vi "Validate Data Types.vi"(8 "error in (no error)":errorcluster, 11 "Cluster":variant) -> (0 "error out":errorcluster)   [LabVIEW 2020, in "MeasurementLink Measurement Server.lvlib"]
uses:
  MeasurementLink Measurement Server.lvlib
  a8e12af1-21a4-44b4-83f7-8cc59a2476b7.vi
  b0d8a33e-d00a-40db-a7bc-a08db774de9e.vi
  <vilib>/Comparison/Equal/Equal Functor/Equal Functor.lvclass
  <vilib>/Utility/Data Type/NI_Data Type.lvlib
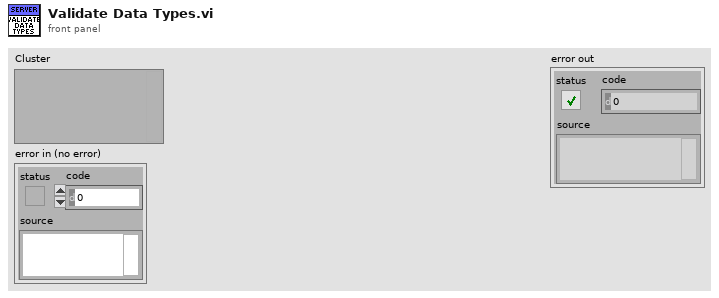
[diagram p1: front panel]
types:
  T1 = typedef "NI_Data Type.lvlib/Data Type.ctl" = enum8{"Invalid Type", "Void", "I8", "I16", "I32", "I64", "U8", "U16", "U32", "U64", "Single Float", "Double Float", "Extended Float", "Single Complex", "Double Complex", "Extended Complex", "Enum U8", "Enum U16", "Enum U32", "Enum U64", "Single Float With Unit", "Double Float With Unit", "Extended Float With Unit", "Single Complex with Unit", "Double Complex with Unit", "Extended Complex with Unit", "Boolean", "String", "Path", "Picture", "Tag", "Array", "Cluster", "Variant", "LV Variant", "Waveform", "Timestamp", "Digital Waveform", "Digital Data", "ExpressData", "Refnum", "External Data", "VI", "Poly VI", "LabVIEW Class Instance", "Fixed Point", "Set Collection", "Map Collection"}
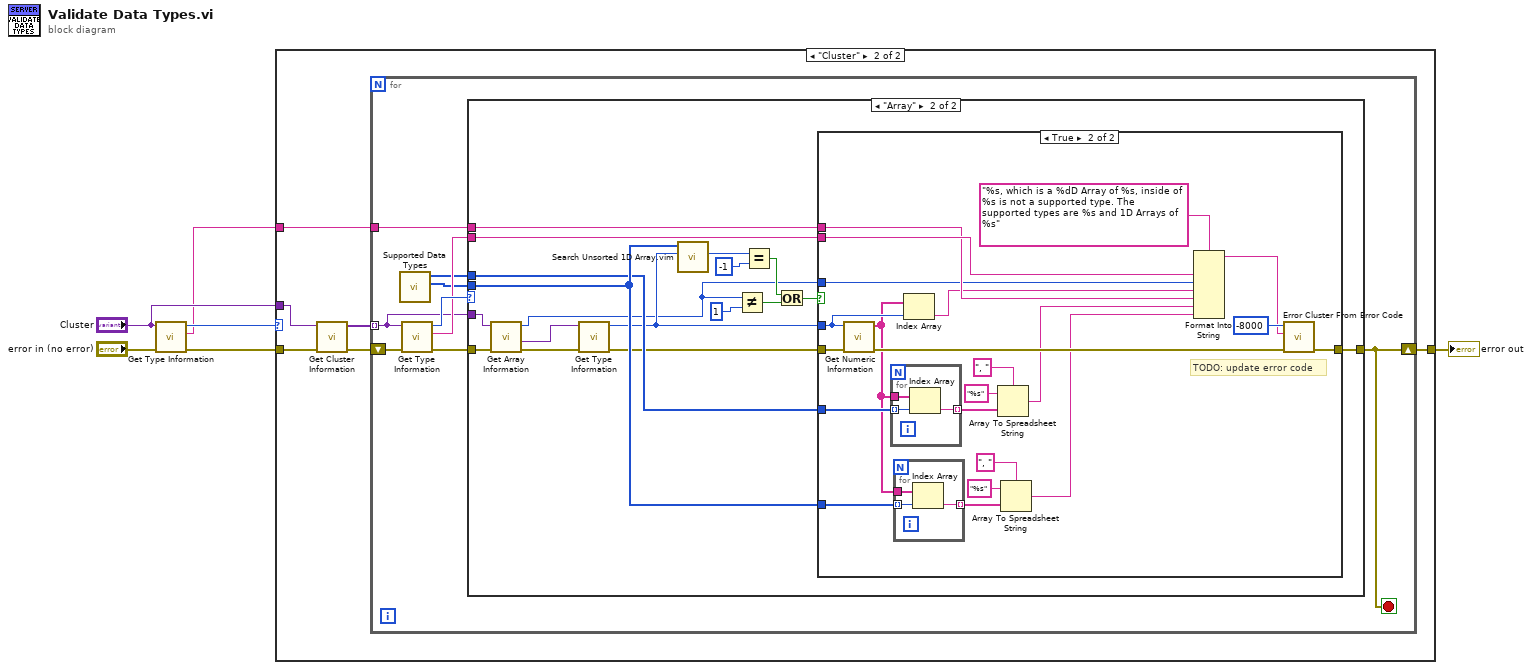
[diagram p0: block diagram]
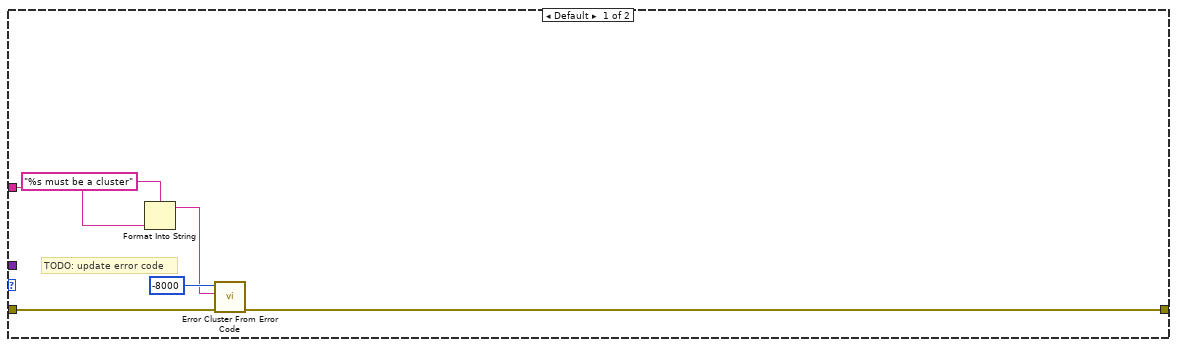
[diagram p2: hidden frame]
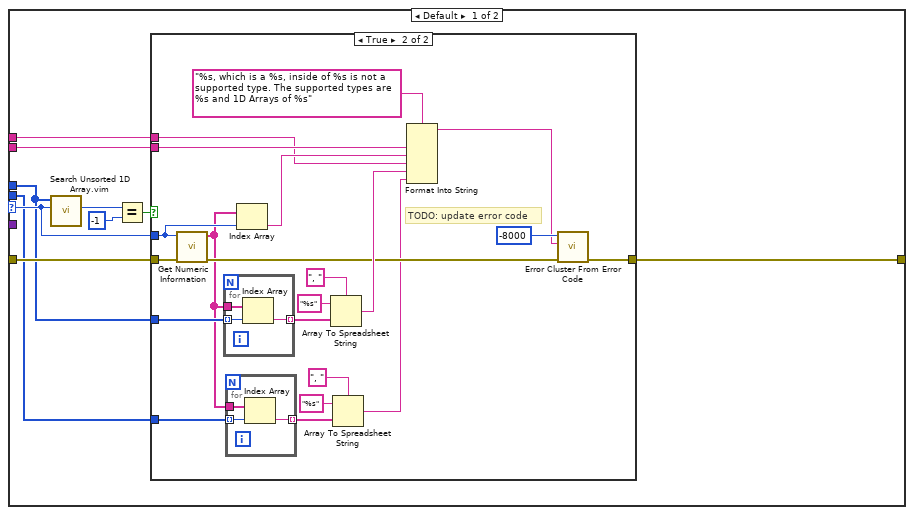
[diagram p3: hidden frame]
diagram:
  n1 = call <vilib>:"Get Type Information.vi"("error in (no error)"="error in (no error)", "variant"="Cluster") -> ("error out"=w6:errorcluster, "name"=w3:string, "type"=w5:T1)  [unwired: 5 in, 2 out]
  n2 = case shown="\"Cluster\"" w5 {
    tunnel: [w11 w13] -> w1
    tunnel: w6 -> [w12 w18]
    tunnel: "Cluster" -> [_ w17]
    tunnel: w3 -> [w8 w14]
    frame Default {
      # "TODO: update error code"
      n3 = Format Into String(format string="%s must be a cluster", w8) -> (resulting string=w7:string)  [unwired: 2 in, 1 out]
      n4 = call <vilib>:"Error Cluster From Error Code.vi"("error in (no error)"=w12, "error message (\"\")"=w7, "error code (0)"=-8000) -> ("error out"=w11:errorcluster)  [unwired: 6 in]
    }
    frame "Cluster" {
      n5 = call <vilib>:"Get Cluster Information.vi"("error in (no error)"=w18, "variant"=w17) -> ("error out"=w16:errorcluster, "cluster elements"=w15:variant[])  [unwired: 8 in]
      n6 = for {
        tunnel: w15 -> [w22] mode=indexing
        tunnel: w14 -> [w25]
        shift-right: [w21] -> w13
        shift-left: w16 -> [w27]
        stop <- w21 stop-if-true
        n7 = call "Supported Data Types.vi"() -> ("Supported Types In Arrays"=w19:T1[], "Supported Types"=w20:T1[])  [unwired: 10 in]
        n8 = call <vilib>:"Get Type Information.vi"("error in (no error)"=w27, "variant"=w22) -> ("error out"=w23:errorcluster, "name"=w24:string, "type"=w26:T1)  [unwired: 5 in, 2 out]
        n9 = case shown="\"Array\"" w26 {
          selector: w26 -> [w33 _]
          tunnel: w20 -> [w31 w71]
          tunnel: w25 -> [w32 w80]
          tunnel: w24 -> [w35 w81]
          tunnel: w23 -> [w34 w77]
          tunnel: [w29 w79] -> w21
          tunnel: w19 -> [w28 w78]
          tunnel: w22 -> [_ w76]
          frame Default {
            n10 = call "Search Unsorted 1D Array.vim"("element"=w33, "unsorted 1D array"=w31) -> ("index of element"=w37:i32)  [unwired: 9 in]
            n11 = Equal?(x=w37, y=-1) -> (x = y?=w30:bool)
            n12 = case shown="True" w30 {
              tunnel: w35 -> [_ w58]
              tunnel: w34 -> [w38 w57]
              tunnel: w33 -> [_ w56]
              tunnel: w32 -> [_ w54]
              tunnel: w31 -> [_ w53]
              tunnel: [w38 w46] -> w29
              tunnel: w28 -> [_ w40]
              frame False {
              }
              frame True {
                # "TODO: update error code"
                n13 = call <vilib>:"Get Numeric Information.vi"("error in (no error)"=w57, "variant"=w56) -> ("error out"=w47:errorcluster, "enum names"=w41:string[])  [unwired: 6 in, 2 out]
                n14 = for {
                  tunnel: w53 -> [w64] mode=indexing
                  tunnel: w41 -> [w65]
                  tunnel: [w63] -> w52 mode=indexing
                  n15 = Index Array(array=w65, index=w64) -> (element=w63:string)
                }
                n16 = for {
                  tunnel: w40 -> [w61] mode=indexing
                  tunnel: w41 -> [w62]
                  tunnel: [w60] -> w42 mode=indexing
                  n17 = Index Array(array=w62, index=w61) -> (element=w60:string)
                }
                n18 = Index Array(array=w41, index=w56) -> (element=w55:string)
                n19 = Array To Spreadsheet String(delimiter (Tab)=", ", array=w52, 3:"%s" ("format string")) -> (spreadsheet string=w49:string)
                n20 = Array To Spreadsheet String(delimiter (Tab)=", ", array=w42, 3:"%s" ("format string")) -> (spreadsheet string=w39:string)
                n21 = Format Into String(format string="%s, which is a %s, inside of %s is not a supported type. The supported types are %s and 1D Arrays of %s", w58, w55, w54, w49, w39) -> (resulting string=w45:string)  [unwired: 2 in, 1 out]
                n22 = call <vilib>:"Error Cluster From Error Code.vi"("error in (no error)"=w47, "error message (\"\")"=w45, "error code (0)"=-8000) -> ("error out"=w46:errorcluster)  [unwired: 6 in]
              }
            }
          }
          frame "Array" {
            n23 = call <vilib>:"Get Array Information.vi"("error in (no error)"=w77, "variant"=w76) -> ("error out"=w70:errorcluster, "array element data type"=w69:variant, "number of dimensions"=w66:i32)  [unwired: 6 in, 1 out]
            n24 = call <vilib>:"Get Type Information.vi"("error in (no error)"=w70, "variant"=w69) -> ("error out"=w68:errorcluster, "type"=w67:T1)  [unwired: 5 in, 3 out]
            n25 = call "Search Unsorted 1D Array.vim"("element"=w67, "unsorted 1D array"=w78) -> ("index of element"=w83:i32)  [unwired: 9 in]
            n26 = Not Equal?(x=w66, y=1) -> (x != y?=w73:bool)
            n27 = Equal?(x=w83, y=-1) -> (x = y?=w74:bool)
            n28 = Or(x=w74, y=w73) -> (x .or. y?=w72:bool)
            n29 = case shown="True" w72 {
              tunnel: w81 -> [_ w105]
              tunnel: w68 -> [w84 w104]
              tunnel: w67 -> [_ w103]
              tunnel: w80 -> [_ w94]
              tunnel: w78 -> [_ w88]
              tunnel: [w84 w98] -> w79
              tunnel: w66 -> [_ w92]
              tunnel: w71 -> [_ w87]
              frame False {
              }
              frame True {
                # "TODO: update error code"
                n30 = call <vilib>:"Get Numeric Information.vi"("error in (no error)"=w104, "variant"=w103) -> ("error out"=w99:errorcluster, "enum names"=w86:string[])  [unwired: 6 in, 2 out]
                n31 = for {
                  tunnel: w87 -> [w111] mode=indexing
                  tunnel: w86 -> [w112]
                  tunnel: [w110] -> w102 mode=indexing
                  n32 = Index Array(array=w112, index=w111) -> (element=w110:string)
                }
                n33 = for {
                  tunnel: w88 -> [w108] mode=indexing
                  tunnel: w86 -> [w109]
                  tunnel: [w107] -> w91 mode=indexing
                  n34 = Index Array(array=w109, index=w108) -> (element=w107:string)
                }
                n35 = Index Array(array=w86, index=w103) -> (element=w93:string)
                n36 = Array To Spreadsheet String(delimiter (Tab)=", ", array=w102, 3:"%s" ("format string")) -> (spreadsheet string=w95:string)
                n37 = Array To Spreadsheet String(delimiter (Tab)=", ", array=w91, 3:"%s" ("format string")) -> (spreadsheet string=w85:string)
                n38 = Format Into String(format string="%s, which is a %dD Array of %s, inside of %s is not a supported type. The supported types are %s and 1D Arrays of %s", w105, w92, w93, w94, w95, w85) -> (resulting string=w96:string)  [unwired: 2 in, 1 out]
                n39 = call <vilib>:"Error Cluster From Error Code.vi"("error in (no error)"=w99, "error message (\"\")"=w96, "error code (0)"=-8000) -> ("error out"=w98:errorcluster)  [unwired: 6 in]
              }
            }
          }
        }
      }
    }
  }
  "error out" <- w1
